vi "ProyectoFinal_PosicionFireBase_SAD.vi"() -> ()   [LabVIEW 2025]
uses:
  <vilib>/httpClient/PUTBuffer.vi
  <vilib>/httpClient/LabVIEWHTTPClient.lvlib
panel:
  out "Error":dbl
  out "error out":errorcluster
  out "Heartbeat":dbl
  out "Posicion":dbl
  out "Fuera de linea":bool
  out "Grafica del Error":dbl(graph)
  in  "stop":bool
  in  "Ganancias":T1
  # "Instituto Politécnico Nacional\nUnidad Profesional Interdisciplinaria de Ingeniería Campus Zacatecas"
  # "Ingeniería en Mecatrónica"
  # "Nodo de Control de Posición vía Firebase"
  # "Desarrollado por:\n- Diego Perez Dominguez\n- Daniel Salas Serna\n- Daniel Acevedo Caldera"
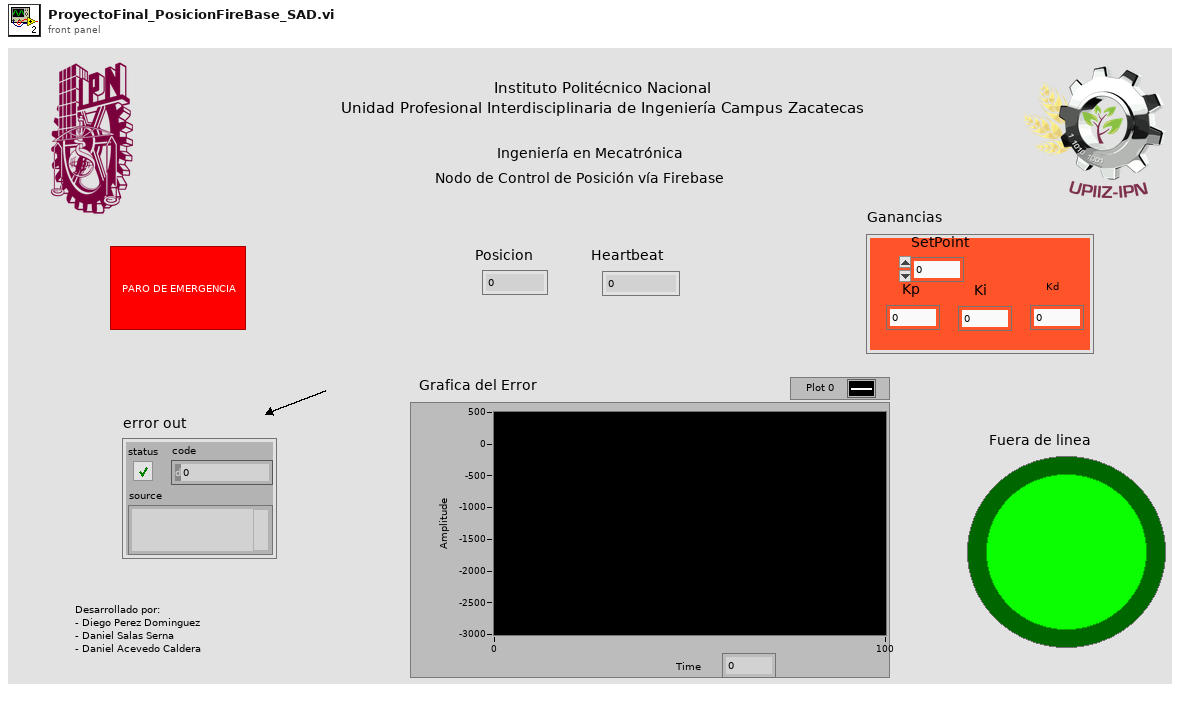
[diagram p1: front panel]
types:
  T1 = cluster{"SetPoint":dbl, "Kp":dbl, "Ki":dbl, "Kd":dbl}
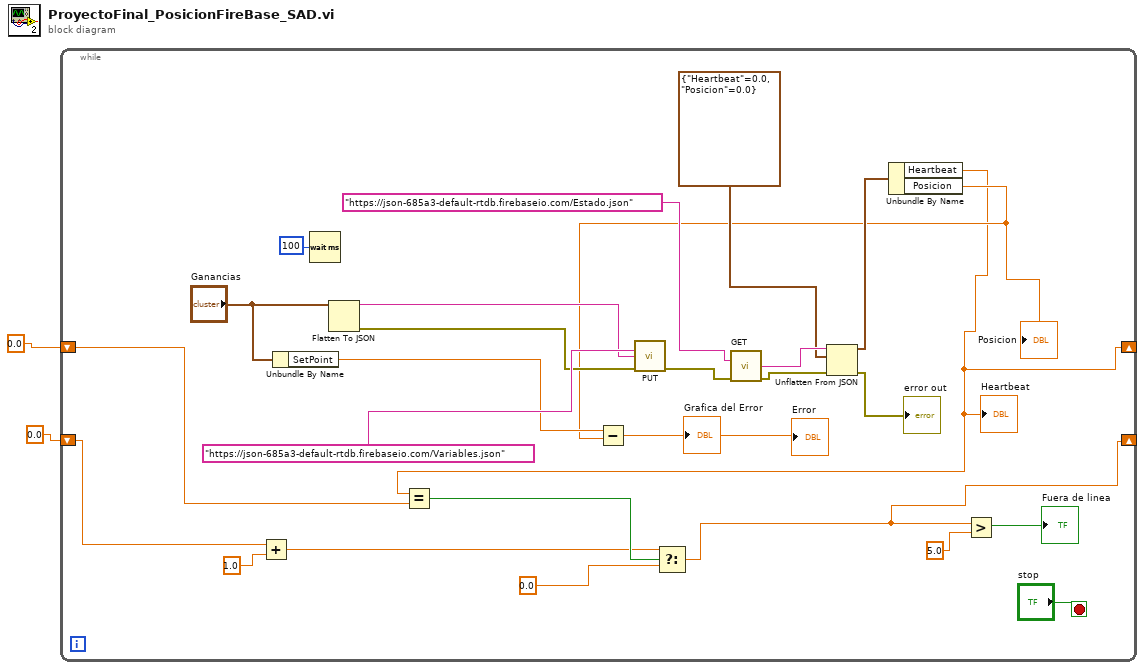
[diagram p0: block diagram]
diagram:
  n1 = while {
    shift-right: [w3] -> _
    shift-left: 0.0 ("x") -> [w17]
    shift-right: [w11] -> _
    shift-left: 0.0 ("x") -> [w14]
    stop <- "stop" stop-if-true
    n2 = Add(x=w14, y=1.0) -> (x+y=w5:dbl)
    n3 = Unbundle By Name("Ganancias") -> ("SetPoint"=w19:dbl)
    n4 = Wait (ms)(milliseconds to wait=u32 100) -> ()  [unwired: 1 out]
    n5 = Flatten To JSON(anything="Ganancias") -> (JSON string=w25:string, 11:w26:errorcluster)  [unwired: 2 in]
    n6 = call-poly <vilib>:"PUT.vi"("url"="https://json-685a3-default-rtdb.firebaseio.com/Variables.json", "buffer"=w25, "error in (no error)"=w26) -> ("error out"=w24:errorcluster)  [unwired: 9 in, 3 out]
    n7 = call <vilib>:"GET.vi"("url"="https://json-685a3-default-rtdb.firebaseio.com/Estado.json", "error in (no error)"=w24) -> ("body"=w22:string, "error out"=w9:errorcluster)  [unwired: 10 in, 2 out]
    n8 = Unflatten From JSON(JSON string=w22, type and defaults=cluster{"Heartbeat":dbl, "Posicion":dbl} {"Heartbeat"=0.0, "Posicion"=0.0}, error in (no error)=w9) -> (value=w7:cluster{"Heartbeat":dbl, "Posicion":dbl}, error out=→"error out":errorcluster)  [unwired: 4 in]
    n9 = Unbundle By Name(w7) -> ("Heartbeat"=w3:dbl, "Posicion"=w6:dbl)
    "Posicion" <- w6
    "Heartbeat" <- w3
    n10 = Equal?(x=w3, y=w17) -> (x = y?=w15:bool)
    n11 = Subtract(x=w19, y=w6) -> (x-y=→"Grafica del Error" →"Error":dbl)
    n12 = Select(t=w5, s=w15, f=0.0) -> (s? t:f=w11:dbl)
    n13 = Greater?(x=w11, y=5.0 ("x")) -> (0:→"Fuera de linea":bool)
  }
